vi "Set Scroll Bar State.vi"(8 "error in (no error)":errorcluster, 10 "Horizontal Scrollbar Visibility":T1(ring), 11 "Pane in":refnum<vi>) -> (0 "error out":errorcluster, 3 "Pane out":refnum<vi>)   [LabVIEW 2015]
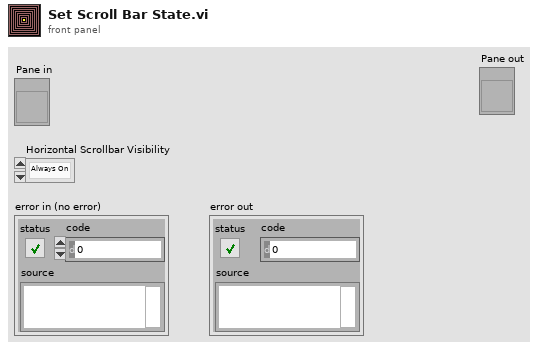
[diagram p1: front panel]
types:
  T1 = enum16{"Always On", "Always Off", "Off While Running"}
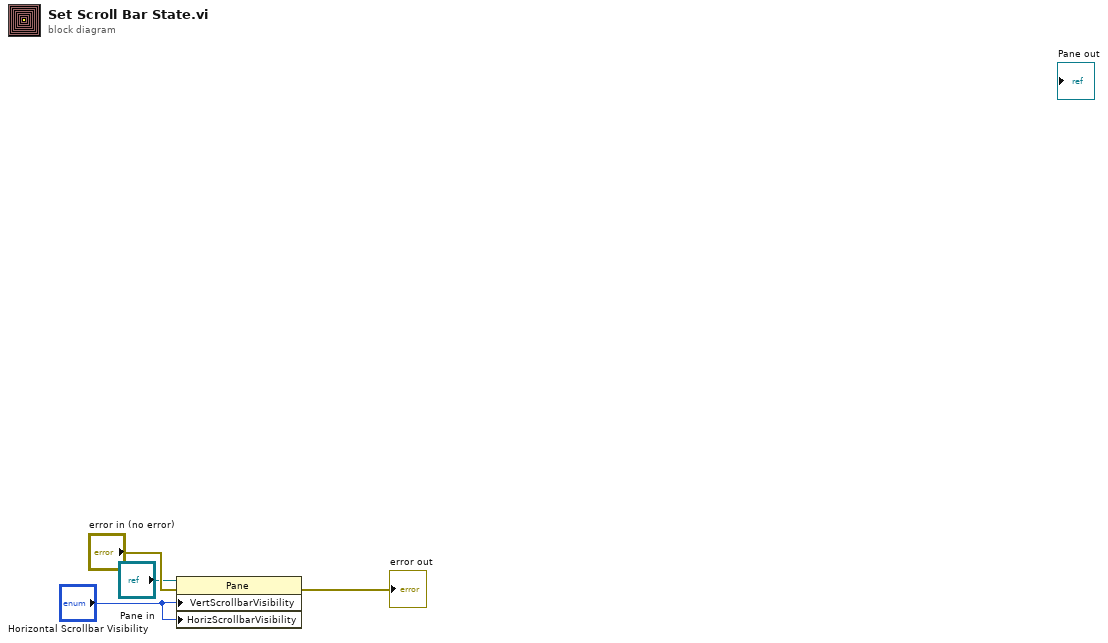
[diagram p0: block diagram]
diagram:
  n1 = property on="Property Node" class="Pane"(reference="Pane in", error in="error in (no error)", "VertScrollbarVisibility"="Horizontal Scrollbar Visibility", "HorizScrollbarVisibility"="Horizontal Scrollbar Visibility") -> (error out=→"error out":errorcluster)  [unwired: 1 out]
